vi "overlay_spots_on_image.vi"(2 "Bubble Size":dbl, 4 "error in":errorcluster, 5 "Selection and Groups":T2[](array[typedef]), 6 "Spots":T3[](array[typedef]) {"Amplitude Correction" step=0.1; "Line Trapping"."Phase Gradient" step=0.05; "Line Trapping"."Vector"."x" step=1e-06 format="%#_6p"; "Line Trapping"."Vector"."y" step=1e-06 format="%#_6p"; "Line Trapping"."Vector"."z" step=1e-06 format="%#_6p"; "NA Position"."r" step=1e-06; "NA Position"."y" step=1e-06; "NA Position"."x" step=1e-06; "Position"."z" step=1e-06; "Position"."y" step=1e-06; "Position"."x" step=1e-06; "Phase" step=0.7753; "Intensity" step=0.1}, 7 "image":T1) -> (0 "error out":errorcluster, 3 "Image":T1(plugin-control))   [LabVIEW 2019]
uses:
  <vilib>/vision/Image Controls.llb/IMAQ Image.ctl
  spot.ctl
  line_trapping.ctl
  selection_element.ctl
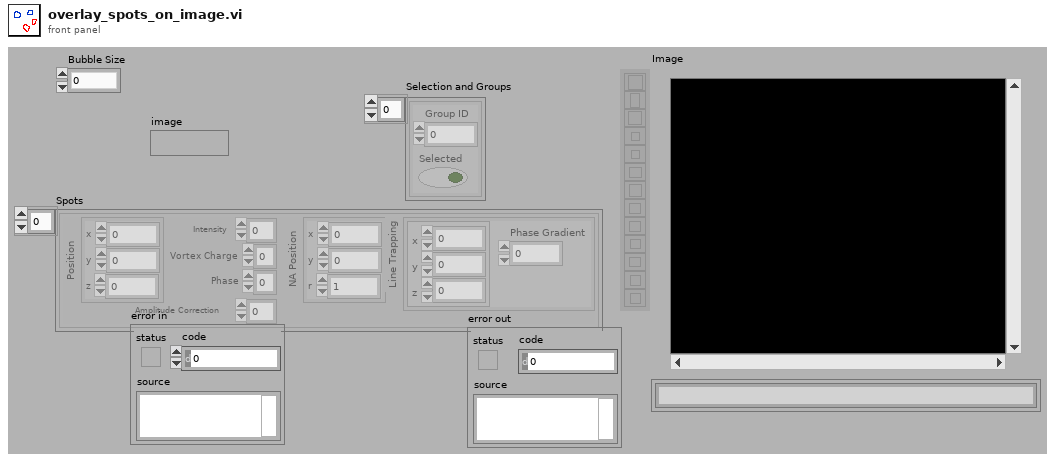
[diagram p1: front panel]
types:
  T1 = typedef "IMAQ Image.ctl" = refnum<image>
  T2 = typedef "selection_element.ctl" = cluster{"Group ID":i32, "Selected":bool}
  T3 = typedef "spot.ctl" = cluster{"Position":cluster{"x":dbl, "y":dbl, "z":dbl}, "Intensity":dbl, "Vortex Charge":i8, "Phase":dbl, "NA Position":cluster{"x":dbl, "y":dbl, "r":dbl}, "Line Trapping":T4, "Amplitude Correction":dbl}
  T4 = typedef "line_trapping.ctl" = cluster{"Vector":cluster{"x":dbl, "y":dbl, "z":dbl}, "Phase Gradient":dbl}
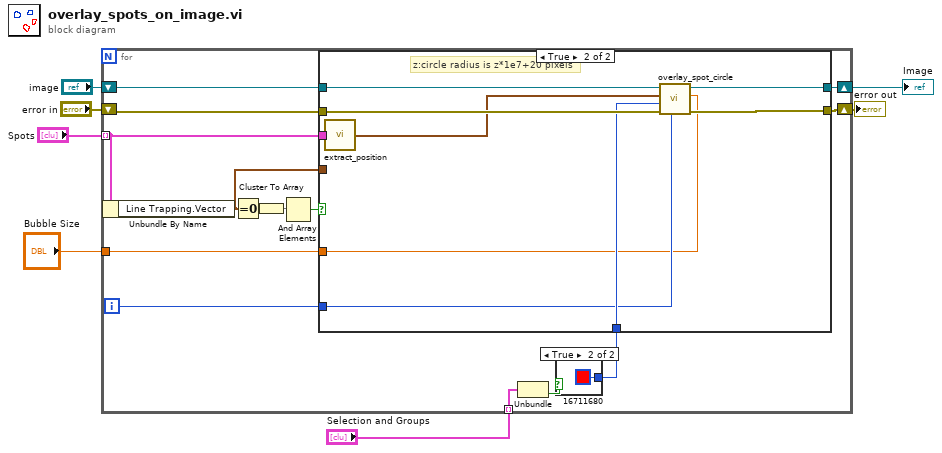
[diagram p0: block diagram]
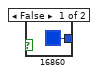
[diagram p2: hidden frame]
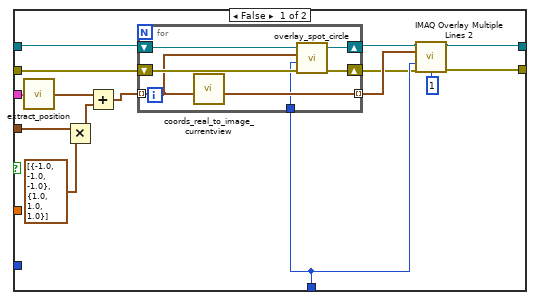
[diagram p3: hidden frame]
diagram:
  n1 = for {
    shift-right: [w20] -> w4
    shift-left: "image" -> [w21]
    tunnel: "Spots" -> [w19] mode=indexing
    tunnel: "Selection and Groups" -> [w15] mode=indexing
    shift-right: [w10] -> w2
    shift-left: "error in" -> [w11]
    tunnel: "Bubble Size" -> [w8]
    i -> [w9]
    n2 = Unbundle By Name(w19) -> ("Line Trapping.Vector"=w13:cluster{"x":dbl, "y":dbl, "z":dbl})
    n3 = Equal To 0?(x=w13) -> (x = 0?=w18:cluster{"x":bool, "y":bool, "z":bool})
    n4 = Cluster To Array(cluster=w18) -> (array=w12:bool[])
    n5 = And Array Elements(Boolean array=w12) -> (logical AND=w17:bool)
    n6 = Unbundle(w15) -> ("Selected"=w16:bool)  [unwired: 1 out]
    n7 = case shown="True" w16 {
      tunnel: [u32 16860 ("color(black)") u32 16711680 ("color(black)")] -> w14
      frame False {
      }
      frame True {
      }
    }
    n8 = case shown="True" w17 {
      tunnel: w21 -> [w34 w53]
      tunnel: [w31 w48] -> w20
      tunnel: w19 -> [w38 w54]
      tunnel: w13 -> [w32 _]
      tunnel: w14 -> [w28 w49]
      tunnel: w11 -> [w25 w52]
      tunnel: [w24 w51] -> w10
      tunnel: w9 -> [_ w47]
      tunnel: w8 -> [_ w46]
      frame False {
        n9 = call "extract_position.vi"("Spot"=w38) -> ("Position"=w36:cluster{"x":dbl, "y":dbl, "z":dbl})
        n10 = Multiply(x=w32, y=cluster{"[0]":dbl, "[1]":dbl, "[2]":dbl}[] [{"[0]"=-1.0, "[1]"=-1.0, "[2]"=-1.0}, {"[0]"=1.0, "[1]"=1.0, "[2]"=1.0}]) -> (x*y=w35:cluster{dbl, dbl, dbl}[])
        n11 = Add(x=w36, y=w35) -> (x+y=w33:cluster{dbl, dbl, dbl}[])
        n12 = for {
          shift-right: [w44] -> w30
          shift-left: w34 -> [w41]
          tunnel: w33 -> [w40] mode=indexing
          tunnel: w28 -> [w39]
          tunnel: [w45] -> w29 mode=indexing
          shift-right: [w43] -> w26
          shift-left: w25 -> [w42]
          n13 = call "coords_real_to_image_currentview.vi"("Position (real coords)"=w40) -> ("Position (pixels, relative to the top left of the image)"=w45:cluster{dbl, dbl})  [unwired: 7 in, 1 out]
          n14 = call "overlay_spot_circle.vi"("error in"=w42, "color(black)"=w39, "Position"=w40, "image"=w41) -> ("error out"=w43:errorcluster, "Image Out"=w44:T1)  [unwired: 3 in]
        }
        n15 = call "IMAQ Overlay Multiple Lines 2"("Image"=w30, "Line End Points"=w29, "Color"=w28, "error in (no error)"=w26, "Width"=u32 1) -> ("Image Out"=w31:T1, "error out"=w24:errorcluster)  [unwired: 9 in]
      }
      frame True {
        # "z:circle radius is z*1e7+20 pixels"
        n16 = call "extract_position.vi"("Spot"=w54) -> ("Position"=w50:cluster{"x":dbl, "y":dbl, "z":dbl})
        n17 = call "overlay_spot_circle.vi"("Bubble Size"=w46, "ID"=w47, "error in"=w52, "color(black)"=w49, "Position"=w50, "image"=w53) -> ("error out"=w51:errorcluster, "Image Out"=w48:T1)  [unwired: 1 in]
      }
    }
  }
  "Image" <- w4
  "error out" <- w2
